vi "Update.vi"(8 "error in (no error)":errorcluster, 10 "Message in":refnum<class "UpdateMessage.lvclass">, 11 "Waveform in":refnum<class "Waveform.lvclass">) -> (0 "error out":errorcluster, 3 "Waveform out":refnum<class "Waveform.lvclass">)   [LabVIEW 2012, in "Waveform.lvclass"]
doc: "The update method processes the command 'update'. \n\nThe command 'update' is used for receiving new values to be set to the private data of the class. This could be seen as a public set method for setting new parameters to the private class data."
uses:
  Waveform.lvclass
  <vilib>/Distrio/Murmex/UpdateMessage/UpdateMessage.lvclass
  Waveform.lvclass/Waveform.ctl
  <vilib>/Distrio/Murmex/Murmex/Murmex.lvclass
panel:
  # "This method is called when the UPDATE\ntrigger is sent. \n\nOverride this method when your component needs to\nrespond to this trigger. \n\nCall parent for proper implementation"
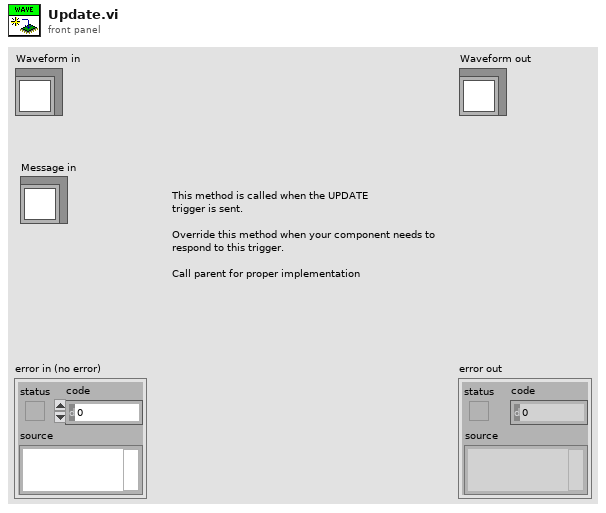
[diagram p1: front panel]
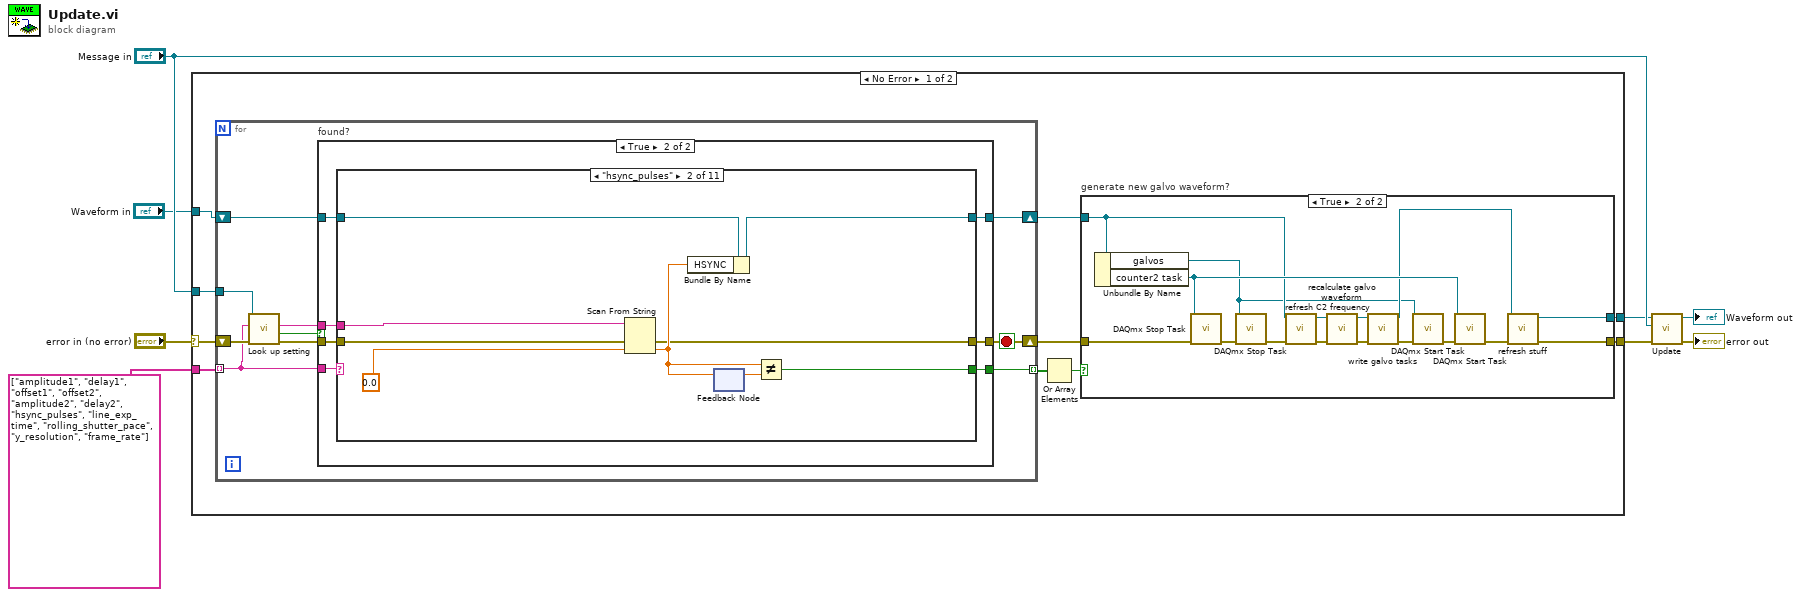
[diagram p0: block diagram]
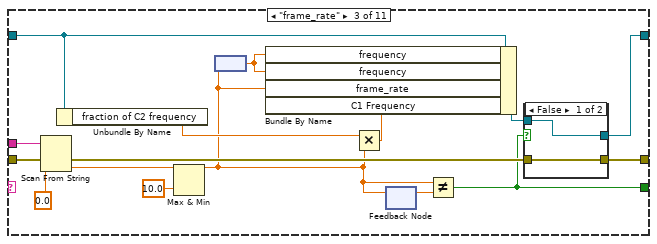
[diagram p5: hidden frame]
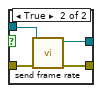
[diagram p6: hidden frame]
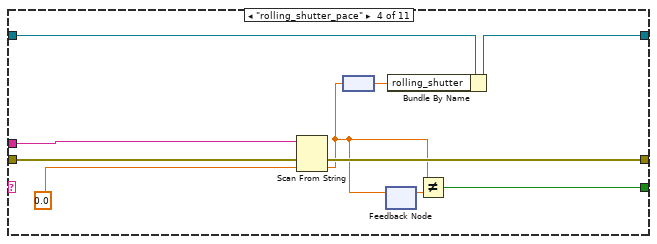
[diagram p7: hidden frame]
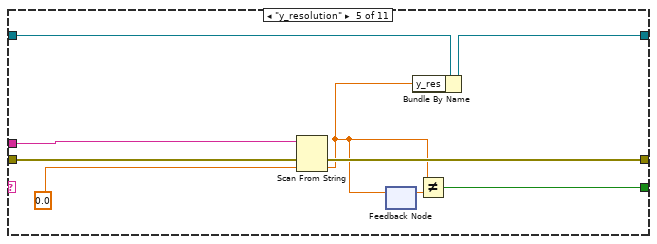
[diagram p8: hidden frame]
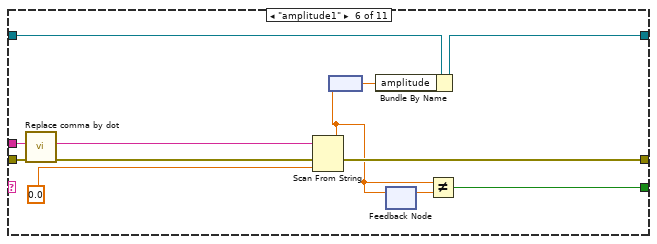
[diagram p9: hidden frame]
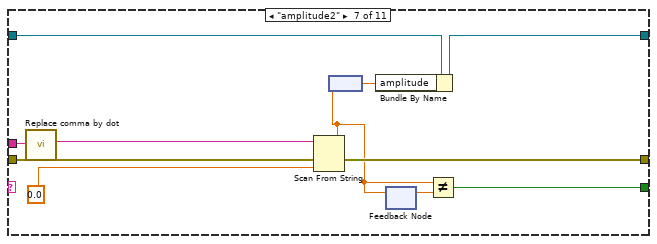
[diagram p10: hidden frame]
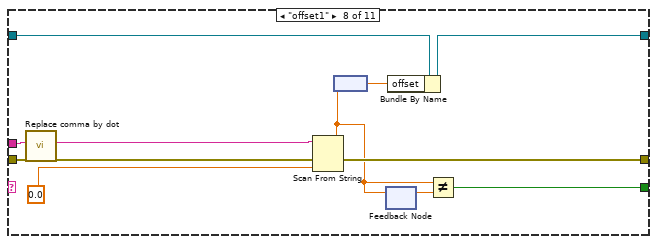
[diagram p11: hidden frame]
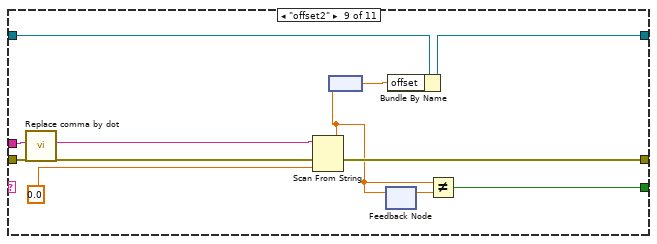
[diagram p12: hidden frame]
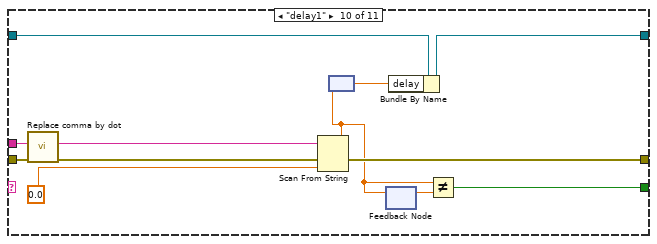
[diagram p13: hidden frame]
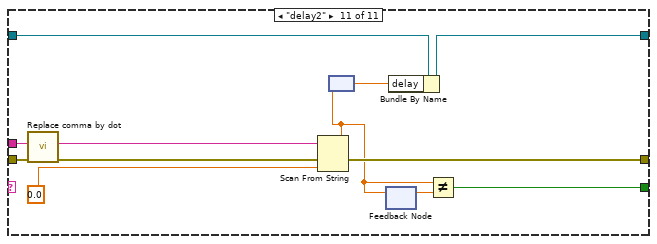
[diagram p14: hidden frame]
diagram:
  n1 = case shown="No Error" "error in (no error)" {
    selector: "error in (no error)" -> [w18 w175]
    tunnel: "Message in" -> [w17 _]
    tunnel: "Waveform in" -> [w16 w176]
    tunnel: string[] ["amplitude1", "delay1", "offset1", "offset2", "amplitude2", "delay2", "hsync_pulses", "line_exp_time", "rolling_shutter_pace", "y_resolution", "frame_rate"] ("key chains") -> [w15 _]
    tunnel: [w11 w175] -> w3
    tunnel: [w10 w176] -> w2
    frame No Error {
      n2 = for {
        shift-right: [w39] -> w12
        shift-left: w18 -> [w46]
        tunnel: w17 -> [w45]
        shift-right: [w40] -> w9
        shift-left: w16 -> [w44]
        tunnel: w15 -> [w37] mode=indexing
        tunnel: [w38] -> w14 mode=indexing
        stop <- w39 stop-if-true
        n3 = call <vilib>:"Look up setting.vi"("error in (no error)"=w46, "tag name"=w37, "UpdateMessage in"=w45) -> ("error out"=w43:errorcluster, "found?"=w42:bool, "value"=w41:string)  [unwired: 5 in, 1 out]
        n4 = case "found?" shown="True" w42 {
          selector: w42 -> [w47 _]
          tunnel: w44 -> [w49 w55]
          tunnel: w43 -> [w48 w56]
          tunnel: w41 -> [_ w51]
          tunnel: w37 -> [_ w53]
          tunnel: [w49 w54] -> w40
          tunnel: [w48 w52] -> w39
          tunnel: [w47 w50] -> w38
          frame False {
          }
          frame True {
            n5 = case shown="\"hsync_pulses\"" w53 {
              tunnel: w56 -> [w57 w67 w83 w99 w108 w119 w130 w141 w152 w163 w174]
              tunnel: w55 -> [w58 w66 w77 w98 w107 w118 w129 w140 w151 w162 w173]
              tunnel: [w58 w60 w72 w97 w106 w117 w128 w139 w150 w161 w172] -> w54
              tunnel: [w57 w59 w74 w96 w105 w116 w127 w138 w149 w160 w171] -> w52
              tunnel: w51 -> [_ w65 w82 w95 w104 w110 w121 w132 w143 w154 w165]
              tunnel: [_ w62 w71 w93 w102 w114 w125 w136 w147 w158 w169] -> w50
              frame Default {
              }
              frame "hsync_pulses" {
                n6 = Scan From String(input string=w65, error in=w67, default 1=0.0) -> (error out=w59:errorcluster, output 1=w63:dbl)  [unwired: 2 in, 2 out]
                n7 = Bundle By Name(cluster=w66, "HSYNC"=w63) -> (w60:refnum<class "Waveform.lvclass">)
                n8 = feedback #1() -> (w64:dbl)  [unwired: 1 in]
                n9 = feedback-in #1(w63) -> ()
                n10 = Not Equal?(x=w63, y=w64) -> (x != y?=w62:bool)
              }
              frame "frame_rate" {
                n11 = Scan From String(input string=w82, error in=w83, default 1=0.0) -> (error out=w75:errorcluster, output 1=w69:dbl)  [unwired: 2 in, 2 out]
                n12 = Unbundle By Name(w77) -> ("fraction of C2 frequency"=w76:dbl)
                n13 = Max & Min(x=w69, y=10.0) -> (max(x,y)=w68:dbl)  [unwired: 1 out]
                n14 = node(w68) -> (w78:dbl[unit])
                n15 = Multiply(x=w76, y=w68) -> (x*y=w79:dbl)
                n16 = Bundle By Name(cluster=w77, "frequency"=w78, "frequency"=w78, "frame_rate"=w68, "C1 Frequency"=w79) -> (w73:refnum<class "Waveform.lvclass">)
                n17 = feedback #2() -> (w81:dbl)  [unwired: 1 in]
                n18 = feedback-in #2(w68) -> ()
                n19 = Not Equal?(x=w68, y=w81) -> (x != y?=w71:bool)
                n20 = case shown="False" w71 {
                  tunnel: w75 -> [w84 w89]
                  tunnel: [w84 w88] -> w74
                  tunnel: w73 -> [w85 w87]
                  tunnel: [w85 w86] -> w72
                  frame False {
                  }
                  frame True {
                    n21 = call-dynamic "send frame rate.vi"("error in (no error)"=w89, "Waveform in"=w87) -> ("error out"=w88:errorcluster, "Waveform out"=w86:refnum<class "Waveform.lvclass">)  [unwired: 8 in]
                  }
                }
              }
              frame "rolling_shutter_pace" {
                n22 = Scan From String(input string=w95, error in=w99, default 1=0.0) -> (error out=w96:errorcluster, output 1=w90:dbl)  [unwired: 2 in, 2 out]
                n23 = node(w90) -> (w91:dbl[unit])
                n24 = feedback #3() -> (w94:dbl)  [unwired: 1 in]
                n25 = feedback-in #3(w90) -> ()
                n26 = Bundle By Name(cluster=w98, "rolling_shutter"=w91) -> (w97:refnum<class "Waveform.lvclass">)
                n27 = Not Equal?(x=w90, y=w94) -> (x != y?=w93:bool)
              }
              frame "y_resolution" {
                n28 = Scan From String(input string=w104, error in=w108, default 1=0.0) -> (error out=w105:errorcluster, output 1=w100:dbl)  [unwired: 2 in, 2 out]
                n29 = feedback #4() -> (w103:dbl)  [unwired: 1 in]
                n30 = feedback-in #4(w100) -> ()
                n31 = Bundle By Name(cluster=w107, "y_res"=w100) -> (w106:refnum<class "Waveform.lvclass">)
                n32 = Not Equal?(x=w100, y=w103) -> (x != y?=w102:bool)
              }
              frame "amplitude1" {
                n33 = call <vilib>:"Replace comma by dot.vi"("input string"=w110) -> ("result string"=w109:string)  [unwired: 10 in]
                n34 = Scan From String(input string=w109, error in=w119, default 1=0.0) -> (error out=w116:errorcluster, output 1=w112:dbl)  [unwired: 2 in, 2 out]
                n35 = node(w112) -> (w113:dbl[unit])
                n36 = Bundle By Name(cluster=w118, "amplitude"=w113) -> (w117:refnum<class "Waveform.lvclass">)
                n37 = feedback #5() -> (w115:dbl)  [unwired: 1 in]
                n38 = feedback-in #5(w112) -> ()
                n39 = Not Equal?(x=w112, y=w115) -> (x != y?=w114:bool)
              }
              frame "amplitude2" {
                n40 = call <vilib>:"Replace comma by dot.vi"("input string"=w121) -> ("result string"=w120:string)  [unwired: 10 in]
                n41 = Scan From String(input string=w120, error in=w130, default 1=0.0) -> (error out=w127:errorcluster, output 1=w123:dbl)  [unwired: 2 in, 2 out]
                n42 = node(w123) -> (w124:dbl[unit])
                n43 = Bundle By Name(cluster=w129, "amplitude"=w124) -> (w128:refnum<class "Waveform.lvclass">)
                n44 = feedback #6() -> (w126:dbl)  [unwired: 1 in]
                n45 = feedback-in #6(w123) -> ()
                n46 = Not Equal?(x=w123, y=w126) -> (x != y?=w125:bool)
              }
              frame "offset1" {
                n47 = call <vilib>:"Replace comma by dot.vi"("input string"=w132) -> ("result string"=w131:string)  [unwired: 10 in]
                n48 = Scan From String(input string=w131, error in=w141, default 1=0.0) -> (error out=w138:errorcluster, output 1=w134:dbl)  [unwired: 2 in, 2 out]
                n49 = node(w134) -> (w135:dbl[unit])
                n50 = feedback #7() -> (w137:dbl)  [unwired: 1 in]
                n51 = feedback-in #7(w134) -> ()
                n52 = Bundle By Name(cluster=w140, "offset"=w135) -> (w139:refnum<class "Waveform.lvclass">)
                n53 = Not Equal?(x=w134, y=w137) -> (x != y?=w136:bool)
              }
              frame "offset2" {
                n54 = call <vilib>:"Replace comma by dot.vi"("input string"=w143) -> ("result string"=w142:string)  [unwired: 10 in]
                n55 = Scan From String(input string=w142, error in=w152, default 1=0.0) -> (error out=w149:errorcluster, output 1=w145:dbl)  [unwired: 2 in, 2 out]
                n56 = node(w145) -> (w146:dbl[unit])
                n57 = feedback #8() -> (w148:dbl)  [unwired: 1 in]
                n58 = feedback-in #8(w145) -> ()
                n59 = Bundle By Name(cluster=w151, "offset"=w146) -> (w150:refnum<class "Waveform.lvclass">)
                n60 = Not Equal?(x=w145, y=w148) -> (x != y?=w147:bool)
              }
              frame "delay1" {
                n61 = call <vilib>:"Replace comma by dot.vi"("input string"=w154) -> ("result string"=w153:string)  [unwired: 10 in]
                n62 = Scan From String(input string=w153, error in=w163, default 1=0.0) -> (error out=w160:errorcluster, output 1=w156:dbl)  [unwired: 2 in, 2 out]
                n63 = node(w156) -> (w157:dbl[unit])
                n64 = feedback #9() -> (w159:dbl)  [unwired: 1 in]
                n65 = feedback-in #9(w156) -> ()
                n66 = Bundle By Name(cluster=w162, "delay"=w157) -> (w161:refnum<class "Waveform.lvclass">)
                n67 = Not Equal?(x=w156, y=w159) -> (x != y?=w158:bool)
              }
              frame "delay2" {
                n68 = call <vilib>:"Replace comma by dot.vi"("input string"=w165) -> ("result string"=w164:string)  [unwired: 10 in]
                n69 = Scan From String(input string=w164, error in=w174, default 1=0.0) -> (error out=w171:errorcluster, output 1=w167:dbl)  [unwired: 2 in, 2 out]
                n70 = node(w167) -> (w168:dbl[unit])
                n71 = feedback #10() -> (w170:dbl)  [unwired: 1 in]
                n72 = feedback-in #10(w167) -> ()
                n73 = Bundle By Name(cluster=w173, "delay"=w168) -> (w172:refnum<class "Waveform.lvclass">)
                n74 = Not Equal?(x=w167, y=w170) -> (x != y?=w169:bool)
              }
            }
          }
        }
      }
      n75 = Or Array Elements(Boolean array=w14) -> (logical OR=w13:bool)
      n76 = case "generate new galvo waveform?" shown="True" w13 {
        tunnel: w12 -> [w19 w34]
        tunnel: [w19 w28] -> w11
        tunnel: [w20 w29] -> w10
        tunnel: w9 -> [w20 w25]
        frame False {
        }
        frame True {
          n77 = Unbundle By Name(w25) -> ("galvos"=w21:refnum<k21>, "counter2 task"=w33:refnum<k21>)
          n78 = call <vilib>:"DAQmx Stop Task.vi"("task/channels in"=w33, "error in"=w34) -> ("error out"=w27:errorcluster)  [unwired: 12 in, 1 out]
          n79 = call <vilib>:"DAQmx Stop Task.vi"("task/channels in"=w21, "error in"=w27) -> ("error out"=w26:errorcluster)  [unwired: 12 in, 1 out]
          n80 = call-dynamic "refresh C2 frequency.vi"("error in (no error)"=w26, "Waveform in"=w25) -> ("error out"=w32:errorcluster, "Waveform out"=w31:refnum<class "Waveform.lvclass">)  [unwired: 8 in]
          n81 = call-dynamic "recalculate galvo waveform.vi"("error in (no error)"=w32, "Waveform in"=w31) -> ("error out"=w36:errorcluster, "Waveform out"=w35:refnum<class "Waveform.lvclass">)  [unwired: 8 in]
          n82 = call-dynamic "write galvo tasks.vi"("error in (no error)"=w36, "Waveform in"=w35) -> ("error out"=w23:errorcluster, "Waveform out"=w22:refnum<class "Waveform.lvclass">)  [unwired: 8 in]
          n83 = call <vilib>:"DAQmx Start Task.vi"("task/channels in"=w21, "error in"=w23) -> ("error out"=w24:errorcluster)  [unwired: 12 in, 1 out]
          n84 = call <vilib>:"DAQmx Start Task.vi"("task/channels in"=w33, "error in"=w24) -> ("error out"=w30:errorcluster)  [unwired: 12 in, 1 out]
          n85 = call-dynamic "refresh stuff.vi"("error in (no error)"=w30, "Waveform in"=w22) -> ("error out"=w28:errorcluster, "Waveform out"=w29:refnum<class "Waveform.lvclass">)  [unwired: 8 in]
        }
      }
    }
    frame Error {
    }
  }
  n86 = call-parent "Update.vi"("error in (no error)"=w3, "Message in"="Message in", "Murmex in"=w2) -> ("error out"=→"error out":errorcluster, "Murmex out"=→"Waveform out":refnum<class "Waveform.lvclass">)  [unwired: 7 in]
